vi "Read Single Value (SubVI).vi"(8 "entrée d'erreur (pas d'erreur)":errorcluster, 11 "Refnum VISA en entrée":refnum<visa-resource-name>) -> (0 "sortie d'erreur":errorcluster, 1 "New data?":bool, 2 "nombre":dbl, 3 "Refnum VISA en sortie":refnum<visa-resource-name>)   [LabVIEW 2017]
doc: "by Tanguy BOULARD"
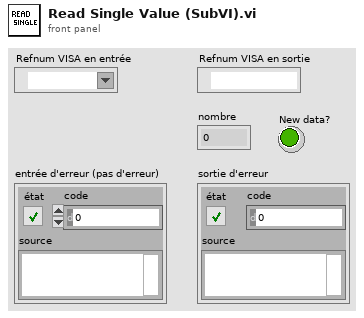
[diagram p1: front panel]
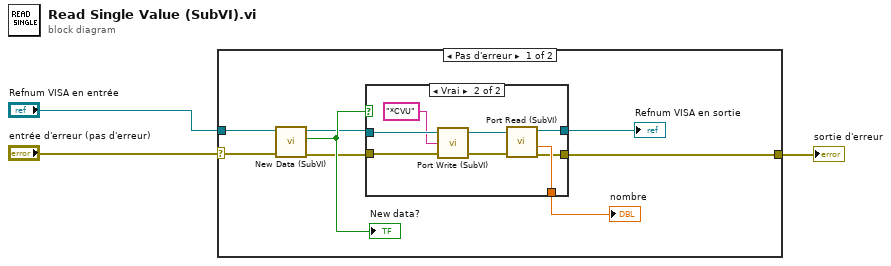
[diagram p0: block diagram]
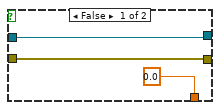
[diagram p2: hidden frame]
diagram:
  n1 = case shown="Pas d'erreur" "entrée d'erreur (pas d'erreur)" {
    selector: "entrée d'erreur (pas d'erreur)" -> [w5 w23]
    tunnel: "Refnum VISA en entrée" -> [w10 _]
    tunnel: [w7 w23] -> w2
    frame No Error {
      n2 = call "New Data (SubVI).vi"("entrée d'erreur (pas d'erreur)"=w5, "Refnum VISA en entrée"=w10) -> ("sortie d'erreur"=w8:errorcluster, "New Data?"=w11:bool, "Refnum VISA en sortie"=w9:refnum<visa-resource-name>)  [unwired: 6 in, 1 out]
      "New data?" <- w11
      n3 = case shown="Vrai" w11 {
        tunnel: w8 -> [w14 w17]
        tunnel: w9 -> [w13 w22]
        tunnel: [0.0 ("nombre") w21] -> w6
        tunnel: [w14 w20] -> w7
        tunnel: [w13 w19] -> w4
        frame False {
        }
        frame True {
          n4 = call "Port Write (SubVI).vi"("error in"=w17, "write buffer"="*CVU", "VISA Refnum in"=w22) -> ("error out"=w16:errorcluster, "VISA Refnum out"=w18:refnum<visa-resource-name>)  [unwired: 1 in]
          n5 = call "Port Read (SubVI).vi"("VISA Refnum in"=w18, "error in"=w16) -> ("VISA Refnum out"=w19:refnum<visa-resource-name>, "nombre"=w21:dbl, "error out"=w20:errorcluster)  [unwired: 1 out]
        }
      }
      "nombre" <- w6
      "Refnum VISA en sortie" <- w4
    }
    frame Error {
    }
  }
  "sortie d'erreur" <- w2
